vi "Get_Device_ID.vi"(8 "错误输入":errorcluster, 11 "枚举":enum16{"电机装配", "ECU装配"}(ring)) -> (0 "错误输出":errorcluster, 3 "Device_ID":string)   [LabVIEW 2020]
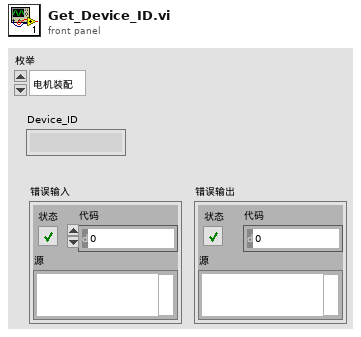
[diagram p1: front panel]
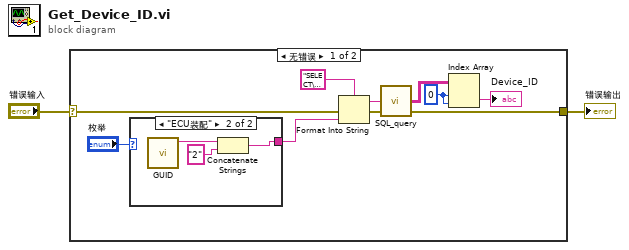
[diagram p0: block diagram]
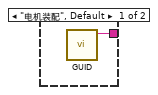
[diagram p2: hidden frame]
diagram:
  n1 = case shown="无错误" "错误输入" {
    selector: "错误输入" -> [w9 w17]
    tunnel: [w7 w17] -> w1
    frame No Error {
      w11 = 0 ("索引 (行)")
      n2 = case shown="\"ECU装配\"" "枚举" {
        tunnel: [w13 w15] -> w3
        frame "电机装配", Default {
          n3 = call "GUID.vi"() -> ("trimmed string"=w13:string)  [unwired: 11 in]
        }
        frame "ECU装配" {
          n4 = call "GUID.vi"() -> ("trimmed string"=w16:string)  [unwired: 11 in]
          n5 = Concatenate Strings(w16, "2" ("字符串")) -> (w15:string)
        }
      }
      n6 = Format Into String(format string="SELECT\ndbo.Device.DEVICE_ID\n\nFROM\ndbo.Device\nWHERE\ndbo.Device.DEVICE_PC_ID = '%s'\n", error in=w9, w3) -> (resulting string=w12:string, error out=w8:errorcluster)  [unwired: 1 in]
      n7 = call "SQL_query.vi"("error in (no error)"=w8, "SQL query"=w12) -> ("error out"=w7:errorcluster, "data"=w6:string[][])  [unwired: 1 in, 1 out]
      n8 = Index Array(array=w6, index (row)=w11, index (col)=w11) -> (element=→"Device_ID":string)
    }
    frame Error {
    }
  }
  "错误输出" <- w1
